vi "palindrome_trial.vi"() -> ()   [LabVIEW 2020]
panel:
  out "Reverse String":string
  out "Palindrome or Not":bool
  in  "Input String":string
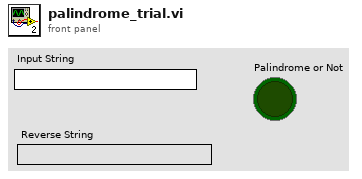
[diagram p1: front panel]
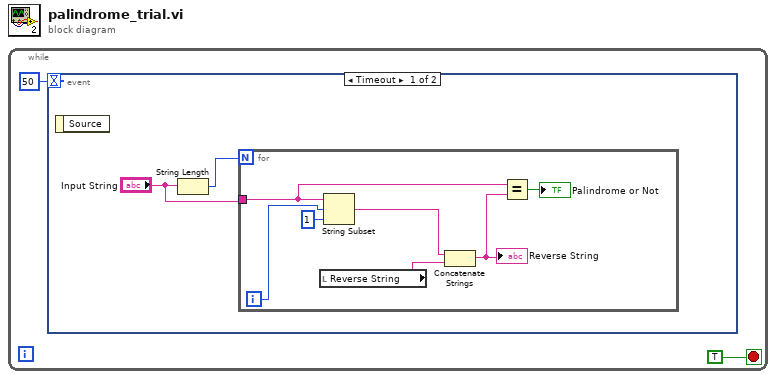
[diagram p0: block diagram]
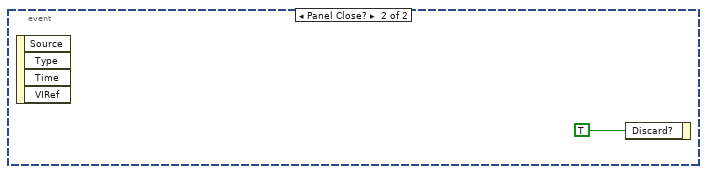
[diagram p2: hidden frame]
diagram:
  n1 = while {
    stop <- TRUE stop-if-true
    n2 = event shown="[0] Timeout" {
      selector: _ -> [_ _]
      dyn-events: _ -> [_ _]
      timeout: 50 -> [_ _]
      event Timeout {
        n3 = event-data() -> ()  [unwired: 1 in, 1 out]
        n4 = String Length(string="Input String") -> (length=w3:i32)
        n5 = for {
          N: w3 -> [_]
          tunnel: "Input String" -> [w7]
          i -> [w8]
          n6 = local read "Reverse String"() -> (w9:string)
          n7 = String Subset(string=w7, offset (0)=w8, length (rest)=1 ("length (rest)")) -> (substring=w10:string)
          n8 = Concatenate Strings(w10, w9) -> (w6:string)
          "Reverse String" <- w6
          n9 = Equal?(x=w7, y=w6) -> (x = y?=→"Palindrome or Not":bool)
        }
      }
      event Panel Close? {
        n10 = event-data() -> ()  [unwired: 1 in, 4 out]
        n11 = event-data("Discard?"=TRUE) -> ()  [unwired: 1 in, 1 out]
      }
    }
  }
